vi "Begin.vi"() -> (0 "error out":errorcluster)   [LabVIEW 2015]
doc: "Called before other user functions, this VI is expected to open initial I/O refnums, load in file data, and do all program initialization. Notice that the <B>error out</B> terminal is simply used for data flow. Wiring it to other structures or subVIs ensures that this VI runs first."
uses:
  <vilib>/Rock Robotics/WPI/DriverStation/WPI_DriverStationRobotMode2.ctl
  Device Refnums.ctl
  <vilib>/Rock Robotics/WPI/Joystick/WPI_JoystickDeviceEnum.ctl
  <vilib>/Rock Robotics/SystemInterfaces/DIO/FPGA_DIOPWMChannel.ctl
  <vilib>/Rock Robotics/WPI/SafetyOutput/WPI_SafetyOutputConfigMenu.ctl
  <vilib>/Rock Robotics/SystemInterfaces/DIO/FPGA_DIOChannel.ctl
  <vilib>/Rock Robotics/WPI/Encoder/WPI_EncoderType.ctl
  <vilib>/Rock Robotics/SystemInterfaces/AI/FPGA_AIChannel.ctl
  <vilib>/Rock Robotics/WPI/CAN/TalonSRX/WPI_CANTalonSRX_APIControlMode.ctl
  <vilib>/Rock Robotics/WPI/Solenoid/WPI_SolenoidChannel.ctl
  Robot Global Data.vi
  <vilib>/Rock Robotics/WPI/Solenoid/WPI_SolenoidOpenSingle.vi
  <vilib>/Rock Robotics/WPI/Solenoid/WPI_SolenoidOpenDouble.vi
  <vilib>/Rock Robotics/WPI/Utilities/WPI_GetSetVariantRefNum.vi
  <vilib>/Rock Robotics/WPI/MotorControl/WPI_MotorControlOpenCANTalonSRX.vi
  <vilib>/Rock Robotics/WPI/Counter/WPI_CounterDigitalInputToDigitalSource.vi
  <vilib>/Rock Robotics/WPI/Switch/WPI_SwitchOpenLimit.vi
  <vilib>/Rock Robotics/WPI/Ultrasonic/WPI_SonarMB1010DigitalOpen.vi
  <vilib>/Rock Robotics/WPI/Ultrasonic/WPI_SonarMB1010DigRefNum Registry Set.vi
  <vilib>/Rock Robotics/WPI/RobotDrive/WPI_RobotDriveOpen2MotorWithSPARK.vi
  <vilib>/Rock Robotics/WPI/MotorControl/WPI_MotorControlOpen VictorSP.vi
  ADIS16448-RoboRIO-Driver/trunk/LabVIEW/ADI MXP IMU/FRC ADI MXP IMU.lvlib
  <vilib>/Rock Robotics/WPI/MotorControl/WPI_MotorControlOpen Victor.vi
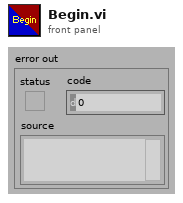
[diagram p1: front panel]
types:
  T1 = typedef "WPI_DriverStationRobotMode2.ctl" = enum16{"Autonomous Disabled", "Autonomous Enabled", "Teleop Disabled", "Teleop Enabled", "Disconnected", "Finish", "Test Disabled", "Test Enabled", "Emergency Stopped"}
  T2 = typedef "WPI_SolenoidChannel.ctl" = enum8{"Solenoid 0", "Solenoid 1", "Solenoid 2", "Solenoid 3", "Solenoid 4", "Solenoid 5", "Solenoid 6", "Solenoid 7", "Invalid"}
  T3 = typedef "Device Refnums.ctl" = string
  T4 = typedef "WPI_SolenoidDevRef.ctl" = cluster{"DevStatus":errorcluster, "Pneumatics Control Module":u8, "Forward Solenoid Channel":T2, "Reverse Solenoid Channel":T2}
  T5 = typedef "WPI_CompressorDevRef.ctl" = cluster{"DevStatus":errorcluster, "Pneumatics Control Module":u8}
  T6 = typedef "WPI_CANTalonSRX_APIControlMode.ctl" = enum8{"Percent VBus", "Speed", "Position", "Slave", "Unchanged / Invalid", "Voltage Compensation", "Current", "Motion Profile"}
  T7 = typedef "WPI_MotorControlDeviceRef.ctl" = cluster{"DeviceStatus":errorcluster, "Type":T8, "PWM":cluster{"PWM Channel":T9, "DeadBand":T10}, "CAN":cluster{"Device Number":u8, "Control Mode":T11, "Semaphore":T12, "Max Vout":dbl, "TalonSRX Control Mode":T6}, "Invert":bool}
  T8 = typedef "WPI_MotorControlType.ctl" = enum16{"PWM", "CAN", "CANTalonSRX"}
  T9 = typedef "FPGA_DIOPWMChannel.ctl" = enum8{"PWM 0", "PWM 1", "PWM 2", "PWM 3", "PWM 4", "PWM 5", "PWM 6", "PWM 7", "PWM 8", "PWM 9", "PWM MXP 0", "PWM MXP 1", "PWM MXP 2", "PWM MXP 3", "PWM MXP 4", "PWM MXP 5", "PWM MXP 6", "PWM MXP 7", "PWM MXP 8", "PWM MXP 9", "Invalid"}
  T10 = typedef "WPI_PWMDeadband.ctl" = cluster{"Name":string, "maxPositivePwm":i32, "minPositivePwm":i32, "centerPwm":i32, "maxNegativePwm":i32, "minNegativePwm":i32, "angularRange":u16}
  T11 = typedef "WPI_CANJaguar_ControlMode.ctl" = enum8{"Percent VBus", "Current", "Speed", "Position", "Voltage"}
  T12 = typedef "Semaphore RefNum" = refnum<k1>
  T13 = typedef "FPGA_AIChannel.ctl" = enum8{"AI 0", "AI 1", "AI 2", "AI 3", "AI MXP 0", "AI MXP 1", "AI MXP 2", "AI MXP 3", "Invalid"}
  T14 = typedef "WPI_AnalogChannelDevRef.ctl" = cluster{"DevStatus":errorcluster, "Analog Channel":T13}
  T15 = typedef "FRC ADI MXP IMU.lvlib/WPI_AnalogDevicesIMUInterruptDevRef.ctl" = cluster{"SimpleGyroDevRef":T16, "InterruptRef":T18}
  T16 = typedef "FRC ADI MXP IMU.lvlib/WPI_AnalogDevicesIMUDevRef.ctl" = cluster{"DevStatus":errorcluster, "Handle":i32, "SPI Bus":T17, "Device Found":bool, "Sample Rate":dbl, "Device Ready":bool, "Yaw Axis":enum16{"X", "Y", "Z"}, "AHRS Algorithm":enum16{"Complementary", "Madgwick"}}
  T17 = typedef "spi_bus.ctl" = enum16{"SPI On-Board, CS0", "SPI On-Board, CS1", "SPI On-Board, CS2", "SPI On-Board, CS3", "SPI MXP", "Invalid"}
  T18 = typedef "WPI_InterruptRef.ctl" = cluster{"DevStatus":errorcluster, "InterruptIndex":T19}
  T19 = typedef "FPGA_InterruptIndex.ctl" = enum8{"0", "1", "2", "3", "4", "5", "6", "7", "Invalid"}
  T20 = typedef "FPGA_DIOChannel.ctl" = enum8{"DIO 0", "DIO 1", "DIO 2", "DIO 3", "DIO 4", "DIO 5", "DIO 6", "DIO 7", "DIO 8", "DIO 9", "DIO MXP 0", "DIO MXP 1", "DIO MXP 2", "DIO MXP 3", "DIO MXP 4", "DIO MXP 5", "DIO MXP 6", "DIO MXP 7", "DIO MXP 8", "DIO MXP 9", "DIO MXP 10", "DIO MXP 11", "DIO MXP 12", "DIO MXP 13", "DIO MXP 14", "DIO MXP 15", "Invalid"}
  T21 = typedef "WPI_EncoderType.ctl" = enum16{"1x", "2x", "4x"}
  T22 = typedef "WPI_SonarMB1010DigitalDeviceRef.ctl" = cluster{"CounterDevRef":T23, "Scaling factor (s/in)":dbl}
  T23 = typedef "WPI_CounterDevRef.ctl" = cluster{"DevStatus":errorcluster, "CntIndex":T24}
  T24 = typedef "FPGA_CounterCtrSystemIndex.ctl" = enum8{"Ctr 0", "Ctr 1", "Ctr 2", "Ctr 3", "Ctr 4", "Ctr 5", "Ctr 6", "Ctr 7", "Invalid"}
  T25 = typedef "WPI_SwitchDevRef.ctl" = cluster{"DevStatus":errorcluster, "DIO Channel":T20, "CntIndex":T24, "Normally Closed":bool}
  T26 = typedef "WPI_DigitalInputDevRef.ctl" = cluster{"DevStatus":errorcluster, "DIO Channel":T20}
  T27 = typedef "FPGA_CounterEncoderSourceConvertionLVSourceType.ctl" = cluster{"DevStatus":errorcluster, "AnalogTriggerMode?":bool, "DigitalMode":cluster{"DIO Channel":T28}, "AnalogTriggerMode":cluster{"AnalogTriggerIndex":T29, "OutputType":T30}}
  T28 = typedef "FPGA_DIODigitalSourceChannel.ctl" = enum8{"DIO 0", "DIO 1", "DIO 2", "DIO 3", "DIO 4", "DIO 5", "DIO 6", "DIO 7", "DIO 8", "DIO 9", "DIO MXP 0", "DIO MXP 1", "DIO MXP 2", "DIO MXP 3", "DIO MXP 4", "DIO MXP 5", "DIO MXP 6", "DIO MXP 7", "DIO MXP 8", "DIO MXP 9", "DIO MXP 10", "DIO MXP 11", "DIO MXP 12", "DIO MXP 13", "DIO MXP 14", "DIO MXP 15", "Disabled"}
  T29 = typedef "FPGA_AnalogTriggerIndex.ctl" = enum8{"Trig 0", "Trig 1", "Trig 2", "Trig 3", "Trig 4", "Trig 5", "Trig 6", "Trig 7", "Invalid"}
  T30 = typedef "FPGA_AnalogTriggerOutType.ctl" = enum16{"InWindow", "TriggerState", "Rising", "Falling"}
  T31 = typedef "WPI_EncoderDevRef.ctl" = cluster{"DevStatus":errorcluster, "EncoderIndex":T32, "CounterIndex":T24, "DistancePerCount":dbl, "Decoding Type":T21}
  T32 = typedef "FPGA_EncoderIdx.ctl" = enum8{"Enc 0", "Enc 1", "Enc 2", "Enc 3", "Enc 4", "Enc 5", "Enc 6", "Enc 7", "Invalid"}
  T33 = typedef "WPI_SafetyOutputConfigMenu.ctl" = enum16{"Enable", "Disable"}
  T34 = typedef "WPI_RobotDriveDevRef.ctl" = cluster{"DevStatus":errorcluster, "Motors[]":T7[], "Square Inputs":bool, "Max Output":dbl}
  T35 = typedef "WPI_JoystickDeviceEnum.ctl" = enum16{"USB 0", "USB 1", "USB 2", "USB 3", "USB 4", "USB 5"}
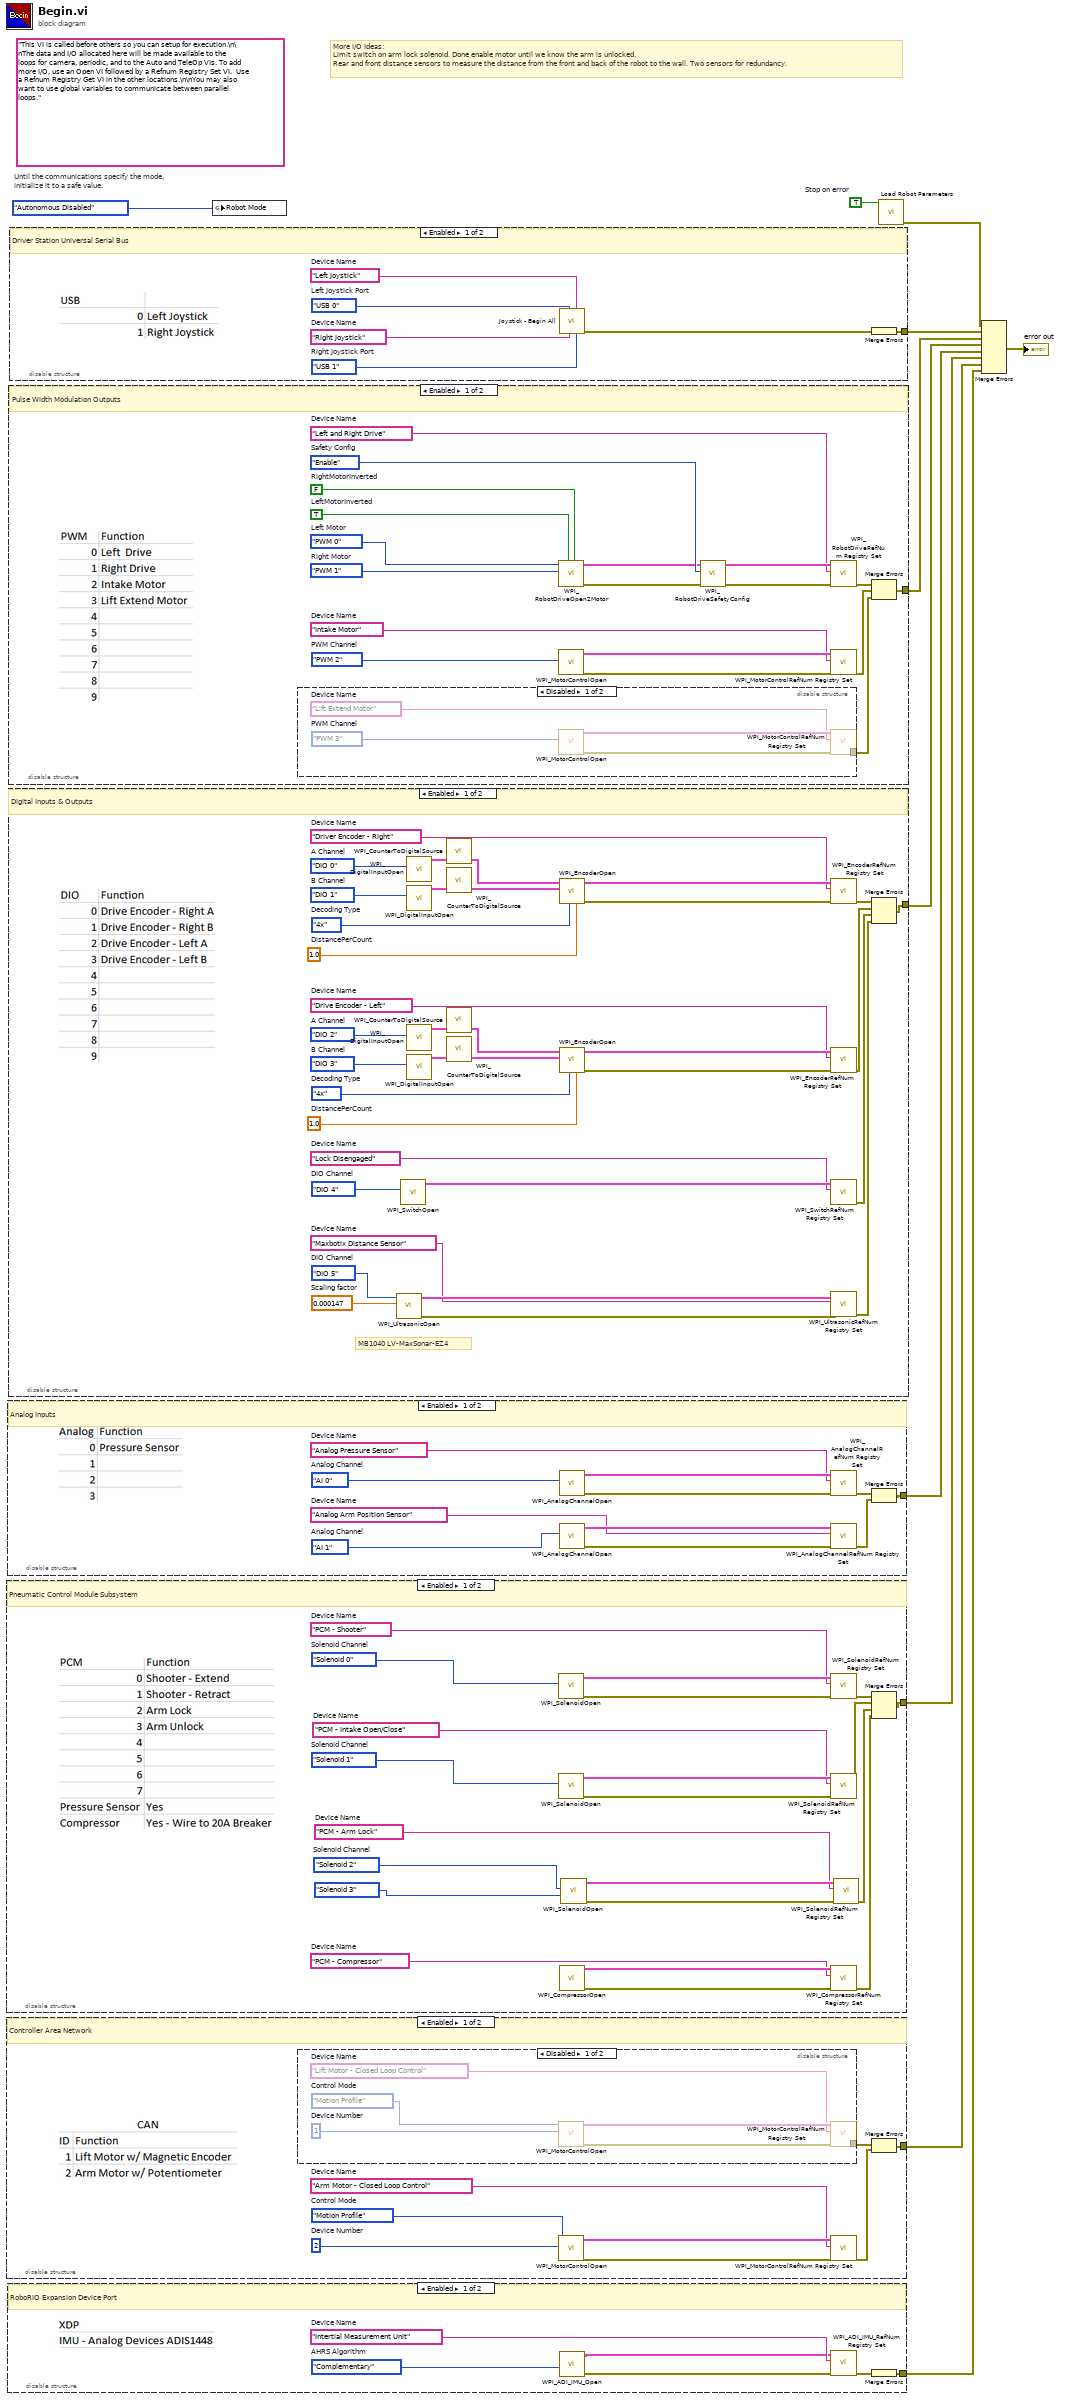
[diagram p0: block diagram]
diagram:
  w2 = TRUE  # Stop on error
  (unwired) "This VI is called before others so you can setup for execution.\n\nThe data and I/O allocated here will be made available to the loops for camera, periodic, and to the Auto and TeleOp VIs. To add more I/O, use an Open VI followed by a Refnum Registry Set VI.  Use a Refnum Registry Get VI in the other locations.\n\nYou may also want to use global variables to communicate between parallel loops."
  # "More I/O Ideas:\nLimit switch on arm lock solenoid. Done enable motor until we know the arm is unlocked.\nRear and front distance sensors to measure the distance from the front and back of the robot to the wall. Two sensors for redundancy."
  # "Until the communications specify the mode,\ninitialize it to a safe value."
  n1 = disable-structure shown="Enabled" {
    disable-tunnel: [w24 _] -> w6
    frame Enabled {
      w13 = T3 "PCM - Intake Open/Close"  # Device Name
      w19 = WPI_SolenoidChannel."Solenoid 2"  # Solenoid Channel
      w20 = T3 "PCM - Compressor"  # Device Name
      w12 = T3 "PCM - Arm Lock"  # Device Name
      w21 = T3 "PCM - Shooter"  # Device Name
      w22 = WPI_SolenoidChannel."Solenoid 0"  # Solenoid Channel
      w23 = WPI_SolenoidChannel."Solenoid 1"  # Solenoid Channel
      # "Pneumatic Control Module Subsystem"
      n2 = call-poly <vilib>:"WPI_SolenoidOpen.vi"("Solenoid Channel"=w22) -> ("error out"=w29:errorcluster, "SolenoidDevRef"=w30:T4)  [unwired: 9 in]
      n3 = call-poly <vilib>:"WPI_SolenoidOpen.vi"("Solenoid Channel"=w23) -> ("error out"=w27:errorcluster, "SolenoidDevRef"=w28:T4)  [unwired: 9 in]
      n4 = call <vilib>:"WPI_CompressorOpen.vi"() -> ("CompressorDevRef"=w31:T5, "error out"=w32:errorcluster)  [unwired: 14 in]
      n5 = call-poly <vilib>:"WPI_SolenoidOpen.vi"("Reverse Solenoid Channel"=WPI_SolenoidChannel."Solenoid 3", "Forward Solenoid Channel"=w19) -> ("error out"=w18:errorcluster, "SolenoidDevRef"=w17:T4)  [unwired: 8 in]
      n6 = call <vilib>:"WPI_SolenoidRefNum Registry Set.vi"("error in (no error)"=w29, "refnum name"=w21, "SolenoidDevRef"=w30) -> ("error out"=w26:errorcluster)  [unwired: 7 in, 1 out]
      n7 = call <vilib>:"WPI_SolenoidRefNum Registry Set.vi"("error in (no error)"=w27, "refnum name"=w13, "SolenoidDevRef"=w28) -> ("error out"=w25:errorcluster)  [unwired: 7 in, 1 out]
      n8 = call <vilib>:"WPI_CompressorRefNum Registry Set.vi"("error in (no error)"=w32, "refnum name"=w20, "CompressorDevRef"=w31) -> ("error out"=w16:errorcluster)  [unwired: 7 in, 1 out]
      n9 = call <vilib>:"WPI_SolenoidRefNum Registry Set.vi"("error in (no error)"=w18, "refnum name"=w12, "SolenoidDevRef"=w17) -> ("error out"=w15:errorcluster)  [unwired: 7 in, 1 out]
      n10 = Merge Errors(w26, w25, w15, w16) -> (w24:errorcluster)
    }
    frame Disabled {
    }
  }
  n11 = disable-structure shown="Enabled" {
    disable-tunnel: [w33 _] -> w5
    frame Enabled {
      w36 = T3 "Arm Motor - Closed Loop Control"  # Device Name
      w37 = u8 2  # Device Number
      w38 = WPI_CANTalonSRX_APIControlMode."Motion Profile"  # Control Mode
      # "Controller Area Network"
      n12 = disable-structure shown="Disabled" {
        disable-tunnel: [w41 _] -> w35
        frame Disabled {
          w42 = T3 "Lift Motor - Closed Loop Control"  # Device Name
          w43 = u8 1  # Device Number
          w44 = WPI_CANTalonSRX_APIControlMode."Motion Profile"  # Control Mode
          n13 = call-poly <vilib>:"WPI_MotorControlOpen.vi"("Device Number"=w43, "Control Mode"=w44) -> ("error out"=w45:errorcluster, "MotorControlDeviceRef"=w46:T7)  [unwired: 8 in]
          n14 = call <vilib>:"WPI_MotorControlRefNum Registry Set.vi"("error in (no error)"=w45, "refnum name"=w42, "MotorControlDevRef"=w46) -> ("error out"=w41:errorcluster)  [unwired: 7 in, 1 out]
        }
        frame Enabled {
        }
      }
      n15 = call-poly <vilib>:"WPI_MotorControlOpen.vi"("Device Number"=w37, "Control Mode"=w38) -> ("error out"=w39:errorcluster, "MotorControlDeviceRef"=w40:T7)  [unwired: 8 in]
      n16 = call <vilib>:"WPI_MotorControlRefNum Registry Set.vi"("error in (no error)"=w39, "refnum name"=w36, "MotorControlDevRef"=w40) -> ("error out"=w34:errorcluster)  [unwired: 7 in, 1 out]
      n17 = Merge Errors(w35, w34) -> (w33:errorcluster)
    }
    frame Disabled {
    }
  }
  n18 = disable-structure shown="Enabled" {
    disable-tunnel: [w53 _] -> w7
    frame Enabled {
      w47 = T3 "Analog Arm Position Sensor"  # Device Name
      w52 = FPGA_AIChannel."AI 1"  # Analog Channel
      w54 = T3 "Analog Pressure Sensor"  # Device Name
      w57 = FPGA_AIChannel."AI 0"  # Analog Channel
      # "Analog Inputs"
      n19 = call <vilib>:"WPI_AnalogChannelOpen.vi"("Analog Channel"=w57) -> ("error out"=w55:errorcluster, "AIDeviceRef"=w56:T14)  [unwired: 9 in]
      n20 = call <vilib>:"WPI_AnalogChannelOpen.vi"("Analog Channel"=w52) -> ("error out"=w51:errorcluster, "AIDeviceRef"=w50:T14)  [unwired: 9 in]
      n21 = call <vilib>:"WPI_AnalogChannelRefNum Registry Set.vi"("error in (no error)"=w55, "refnum name"=w54, "AIDeviceRef"=w56) -> ("error out"=w49:errorcluster)  [unwired: 7 in, 1 out]
      n22 = call <vilib>:"WPI_AnalogChannelRefNum Registry Set.vi"("error in (no error)"=w51, "refnum name"=w47, "AIDeviceRef"=w50) -> ("error out"=w48:errorcluster)  [unwired: 7 in, 1 out]
      n23 = Merge Errors(w49, w48) -> (w53:errorcluster)
    }
    frame Disabled {
    }
  }
  n24 = disable-structure shown="Enabled" {
    disable-tunnel: [w61 _] -> w4
    frame Enabled {
      w63 = T3 "Intertial Measurement Unit"  # Device Name
      w60 = enum16{"Complementary", "Madgwick"}."Complementary"  # AHRS Algorithm
      # "RoboRIO Expansion Device Port"
      n25 = call "WPI_ADI_IMU_Open.vi"("AHRS Algorithm"=w60) -> ("error out"=w58:errorcluster, "ADI IMU Interrupt DevRef"=w59:T15)  [unwired: 9 in]
      n26 = call "WPI_ADI_IMU_RefNum Registry Set.vi"("error in (no error)"=w58, "refnum name"=w63, "ADI IMU Interrupt DevRef"=w59) -> ("error out"=w62:errorcluster)  [unwired: 7 in, 1 out]
      n27 = Merge Errors(w62) -> (w61:errorcluster)
    }
    frame Disabled {
    }
  }
  n28 = disable-structure shown="Enabled" {
    disable-tunnel: [w74 _] -> w8
    frame Enabled {
      w65 = FPGA_DIOChannel."DIO 5"  # DIO Channel
      w66 = 0.000147  # Scaling factor
      w67 = T3 "Maxbotix Distance Sensor"  # Device Name
      w70 = T3 "Lock Disengaged"  # Device Name
      w73 = FPGA_DIOChannel."DIO 4"  # DIO Channel
      w77 = T3 "Drive Encoder - Left"  # Device Name
      w78 = T3 "Driver Encoder - Right"  # Device Name
      w79 = 1.0  # DistancePerCount
      w80 = 1.0  # DistancePerCount
      w81 = WPI_EncoderType."4x"  # Decoding Type
      w82 = WPI_EncoderType."4x"  # Decoding Type
      w85 = FPGA_DIOChannel."DIO 3"  # B Channel
      w86 = FPGA_DIOChannel."DIO 2"  # A Channel
      w93 = FPGA_DIOChannel."DIO 1"  # B Channel
      w94 = FPGA_DIOChannel."DIO 0"  # A Channel
      # "MB1040 LV-MaxSonar-EZ4"
      # "Digital Inputs & Outputs"
      n29 = call-poly <vilib>:"WPI_UltrasonicOpen.vi"("Scaling factor (s/in)"=w66, "DIO Channel"=w65) -> ("error out"=w68:errorcluster, "SonarMB1010DigitalDevRef"=w69:T22)  [unwired: 8 in]
      n30 = call-poly <vilib>:"WPI_SwitchOpen.vi"("DIO Channel"=w73) -> ("SwitchDevRef"=w72:T25)  [unwired: 9 in, 1 out]
      n31 = call <vilib>:"WPI_DigitalInputOpen.vi"("DIO Channel"=w94) -> ("DigitalInputDevRef"=w97:T26)  [unwired: 1 in, 9 out]
      n32 = call <vilib>:"WPI_DigitalInputOpen.vi"("DIO Channel"=w93) -> ("DigitalInputDevRef"=w96:T26)  [unwired: 1 in, 9 out]
      n33 = call <vilib>:"WPI_DigitalInputOpen.vi"("DIO Channel"=w86) -> ("DigitalInputDevRef"=w89:T26)  [unwired: 1 in, 9 out]
      n34 = call <vilib>:"WPI_DigitalInputOpen.vi"("DIO Channel"=w85) -> ("DigitalInputDevRef"=w88:T26)  [unwired: 1 in, 9 out]
      n35 = call-poly <vilib>:"WPI_CounterToDigitalSource.vi"("DigitalInputDevRef"=w97) -> ("Digital Source"=w98:T27)  [unwired: 6 out]
      n36 = call-poly <vilib>:"WPI_CounterToDigitalSource.vi"("DigitalInputDevRef"=w96) -> ("Digital Source"=w95:T27)  [unwired: 6 out]
      n37 = call-poly <vilib>:"WPI_CounterToDigitalSource.vi"("DigitalInputDevRef"=w89) -> ("Digital Source"=w90:T27)  [unwired: 6 out]
      n38 = call-poly <vilib>:"WPI_CounterToDigitalSource.vi"("DigitalInputDevRef"=w88) -> ("Digital Source"=w87:T27)  [unwired: 6 out]
      n39 = call <vilib>:"WPI_EncoderOpen.vi"("DistancePerCount"=w80, "Decoding Type"=w81, "BSource"=w95, "ASource"=w98) -> ("error out"=w92:errorcluster, "EncoderDevRef"=w91:T31)  [unwired: 4 in, 2 out]
      n40 = call <vilib>:"WPI_EncoderOpen.vi"("DistancePerCount"=w79, "Decoding Type"=w82, "BSource"=w87, "ASource"=w90) -> ("error out"=w84:errorcluster, "EncoderDevRef"=w83:T31)  [unwired: 4 in, 2 out]
      n41 = call <vilib>:"WPI_EncoderRefNum Registry Set.vi"("error in (no error)"=w92, "refnum name"=w78, "EncoderDevRef"=w91) -> ("error out"=w76:errorcluster)  [unwired: 7 in, 1 out]
      n42 = call <vilib>:"WPI_EncoderRefNum Registry Set.vi"("error in (no error)"=w84, "refnum name"=w77, "EncoderDevRef"=w83) -> ("error out"=w75:errorcluster)  [unwired: 7 in, 1 out]
      n43 = call <vilib>:"WPI_SwitchRefNum Registry Set.vi"("refnum name"=w70, "SwitchDevRef"=w72) -> ("error out"=w71:errorcluster)  [unwired: 8 in, 1 out]
      n44 = call-poly <vilib>:"WPI_UltrasonicRefNum Registry Set.vi"("error in (no error)"=w68, "refnum name"=w67, "SonarMB1010DigitalDevRef"=w69) -> ("error out"=w64:errorcluster)  [unwired: 7 in, 1 out]
      n45 = Merge Errors(w76, w75, w71, w64) -> (w74:errorcluster)
    }
    frame Disabled {
    }
  }
  n46 = disable-structure shown="Enabled" {
    disable-tunnel: [w99 _] -> w9
    frame Enabled {
      w103 = T3 "Intake Motor"  # Device Name
      w104 = T3 "Left and Right Drive"  # Device Name
      w107 = FPGA_DIOPWMChannel."PWM 2"  # PWM Channel
      w112 = WPI_SafetyOutputConfigMenu."Enable"  # Safety Config
      w113 = FPGA_DIOPWMChannel."PWM 1"  # Right Motor
      w114 = FPGA_DIOPWMChannel."PWM 0"  # Left Motor
      w115 = TRUE  # LeftMotorInverted
      w116 = FALSE  # RightMotorInverted
      # "Pulse Width Modulation Outputs"
      n47 = disable-structure shown="Disabled" {
        disable-tunnel: [w117 _] -> w101
        frame Disabled {
          w118 = T3 "Lift Extend Motor"  # Device Name
          w120 = FPGA_DIOPWMChannel."PWM 3"  # PWM Channel
          n48 = call-poly <vilib>:"WPI_MotorControlOpen.vi"("PWM Channel"=w120) -> ("error out"=w119:errorcluster, "MotorControlDeviceRef"=w121:T7)  [unwired: 9 in]
          n49 = call <vilib>:"WPI_MotorControlRefNum Registry Set.vi"("error in (no error)"=w119, "refnum name"=w118, "MotorControlDevRef"=w121) -> ("error out"=w117:errorcluster)  [unwired: 7 in, 1 out]
        }
        frame Enabled {
        }
      }
      n50 = call-poly <vilib>:"WPI_RobotDriveOpen2Motor.vi"("Right Motor Inverted"=w116, "Left Motor Inverted"=w115, "Right Motor"=w113, "Left Motor"=w114) -> ("error out"=w109:errorcluster, "RobotDriveDevRef"=w108:T34)  [unwired: 1 in, 5 out]
      n51 = call-poly <vilib>:"WPI_MotorControlOpen.vi"("PWM Channel"=w107) -> ("error out"=w105:errorcluster, "MotorControlDeviceRef"=w106:T7)  [unwired: 9 in]
      n52 = call <vilib>:"WPI_RobotDriveSafetyConfig.vi"("error in (no error)"=w109, "mode"=w112, "RobotDriveDevRef"=w108) -> ("error out"=w111:errorcluster, "RobotDriveDevRef"=w110:T34)  [unwired: 7 in]
      n53 = call <vilib>:"WPI_RobotDriveRefNum Registry Set.vi"("error in (no error)"=w111, "refnum name"=w104, "RobotDriveDevRef"=w110) -> ("error out"=w102:errorcluster)  [unwired: 1 in, 7 out]
      n54 = call <vilib>:"WPI_MotorControlRefNum Registry Set.vi"("error in (no error)"=w105, "refnum name"=w103, "MotorControlDevRef"=w106) -> ("error out"=w100:errorcluster)  [unwired: 7 in, 1 out]
      n55 = Merge Errors(w102, w100, w101) -> (w99:errorcluster)
    }
    frame Disabled {
    }
  }
  n56 = disable-structure shown="Enabled" {
    disable-tunnel: [w122 _] -> w10
    frame Enabled {
      w124 = T3 "Right Joystick"  # Device Name
      w125 = T3 "Left Joystick"  # Device Name
      w126 = WPI_JoystickDeviceEnum."USB 1"  # Right Joystick Port
      w127 = WPI_JoystickDeviceEnum."USB 0"  # Left Joystick Port
      # "Driver Station Universal Serial Bus"
      n57 = call "Joystick - Begin All.vi"("Right Joystick Port"=w126, "Left Joystick Name"=w125, "Right Joystick Name"=w124, "Left Joystick Port"=w127) -> ("error out"=w123:errorcluster)  [unwired: 7 in]
      n58 = Merge Errors(w123) -> (w122:errorcluster)
    }
    frame Disabled {
    }
  }
  n59 = global write "Robot Global Data.vi" "Robot Mode"(WPI_DriverStationRobotMode2."Autonomous Disabled" ("Robot Mode")) -> ()
  n60 = call "Load Robot Parameters.vi"("Stop on error"=w2) -> ("error out"=w1:errorcluster)  [unwired: 10 in]
  n61 = Merge Errors(w1, w10, w9, w8, w7, w6, w5, w4) -> (→"error out":errorcluster)
